vi "HC-SR04 Module Test.vi"(2 "Stop Button":bool) -> (0 "output cluster":T1, 1 "CM O/P":cluster{"US FR":sgl, "US FL":sgl, "US BK":sgl})   [LabVIEW 2015]
uses:
  <vilib>/FPGAPlugInAG/myRIO-1900/niLvFpga_Open_myRIO-1900.vi
  <vilib>/rvi/interface/common/dynamic/niFpgaDynamicAddResources.vi
  <vilib>/FPGAPlugInAG/Dynamic/niLvFpga_Run_Dynamic.vi
  <vilib>/FPGAPlugInAG/Dynamic/niLvFpga_Close_Dynamic.vi
  <vilib>/rvi/interface/nirviOpenFPGA/nirviOpenFPGA.xnode
  FPGA Bitfiles/ReconRover_FPGATarget-Wi-Fi_Express2_ln+iIhdshGM.lvbitx
  FPGA/Express.vi
  <vilib>/rvi/interface/nirviMethod/nirviMethod.xnode
  <vilib>/rvi/interface/nirviCloseFPGA/nirviCloseFPGA.xnode
panel:
  in  "Threshold":sgl=2.3
  out "Error Out":errorcluster
  in  "Error In":errorcluster
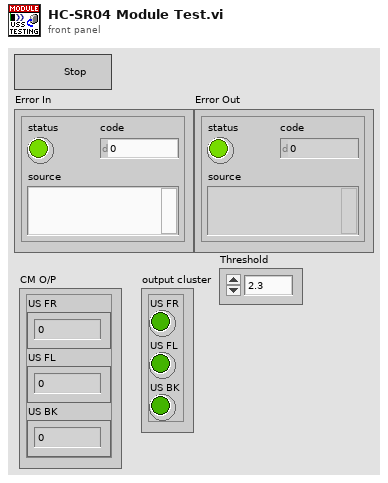
[diagram p1: front panel]
types:
  T1 = cluster{"US FR":bool, "US FL":bool, "US BK":bool}
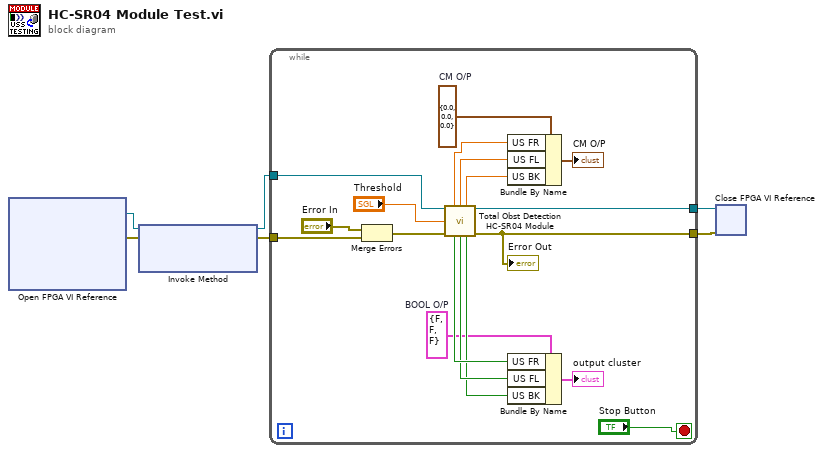
[diagram p0: block diagram]
diagram:
  n1 = xnode "Open FPGA VI Reference"() -> ("FPGA VI Reference Out"=w6:refnum<k20>, "error out"=w5:errorcluster)  [unwired: 2 in]
  n2 = xnode "Invoke Method"("FPGA VI Reference In"=w6, "error in"=w5) -> ("FPGA VI Reference Out"=w1:refnum<k20>, "error out"=w2:errorcluster)  [unwired: 1 in]
  n3 = while {
    tunnel: [w13] -> w4
    tunnel: [w12] -> w3
    tunnel: w2 -> [w10]
    tunnel: w1 -> [w9]
    stop <- "Stop Button" stop-if-true
    w16 = T1 {"US FR"=FALSE, "US FL"=FALSE, "US BK"=FALSE}  # BOOL O/P
    w21 = cluster{"US FR":sgl, "US FL":sgl, "US BK":sgl} {"US FR"=0.0, "US FL"=0.0, "US BK"=0.0}  # CM O/P
    n4 = Merge Errors("Error In", w10) -> (w8:errorcluster)
    n5 = call "Total Obst Detection HC-SR04 Module.vi"("FPGA VI Reference In"=w9, "Threshold"="Threshold", "Error In"=w8) -> (1:"US FR"=w24:sgl, 2:"US FL"=w23:sgl, 3:"US BK"=w22:sgl, "FPGA VI Reference Out"=w13:refnum<k20>, 12:"US FR"=w19:bool, 13:"US FL"=w18:bool, 14:"US BK"=w17:bool, "Error Out"=w12:errorcluster)  [unwired: 5 in]
    "Error Out" <- w12
    n6 = Bundle By Name(cluster=w21, "US FR"=w24, "US FL"=w23, "US BK"=w22) -> (→"CM O/P":cluster{"US FR":sgl, "US FL":sgl, "US BK":sgl})
    n7 = Bundle By Name(cluster=w16, "US FR"=w19, "US FL"=w18, "US BK"=w17) -> (→"output cluster":T1)
  }
  n8 = xnode "Close FPGA VI Reference"("FPGA VI Reference In"=w4, "error in"=w3) -> ()  [unwired: 1 out]
